vi "FTW-STR-Random-UTF8chars.vi"(3 "String Length":i32=32) -> (0 "Random UTF-8 Characters":string)   [LabVIEW 2013]
panel:
  out "Array 2":i32[](array[numeric])
  out "Numeric":i32
  out "Array":string[](array[string])
  out "x/y":dbl
  # "Inputs"
  # "Outputs"
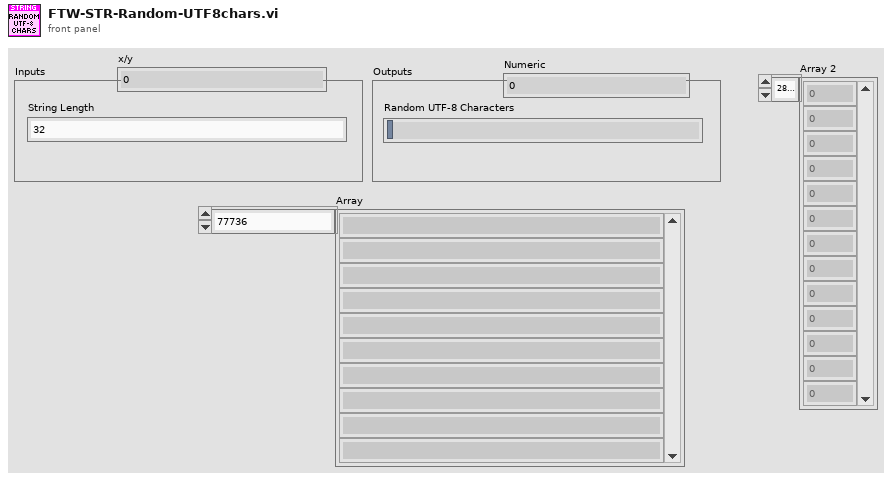
[diagram p1: front panel]
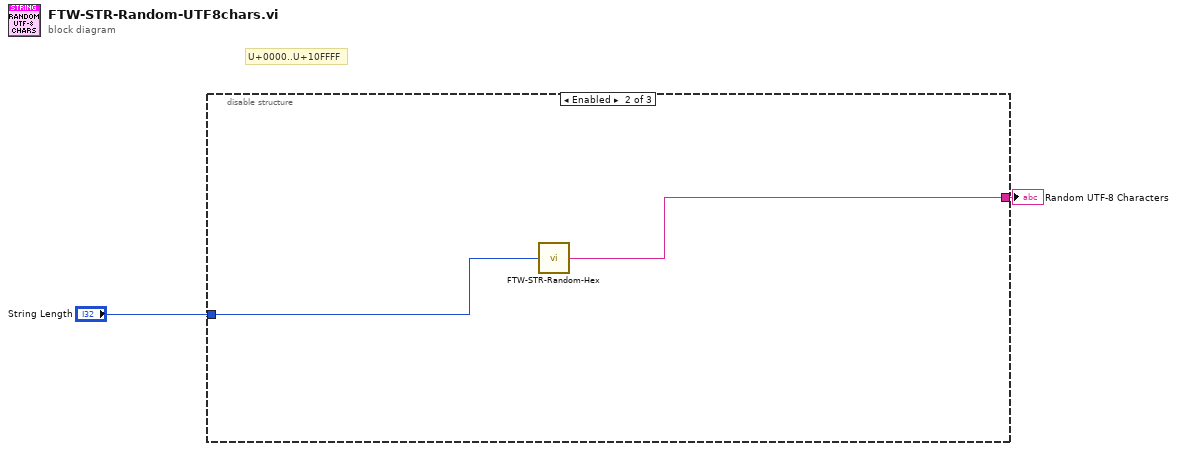
[diagram p0: block diagram]
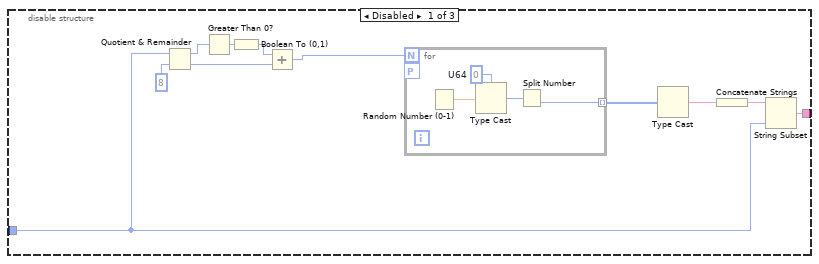
[diagram p2: hidden frame]
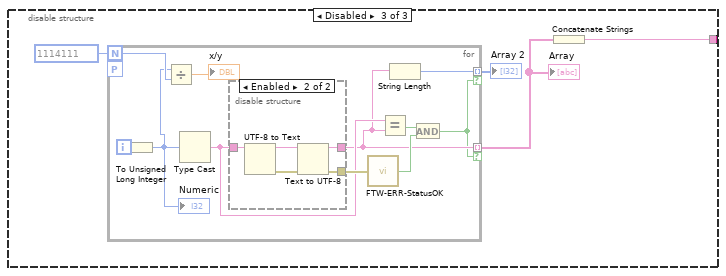
[diagram p3: hidden frame]
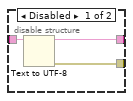
[diagram p4: hidden frame]
diagram:
  # "U+0000..U+10FFFF"
  n1 = disable-structure shown="Enabled" {
    disable-tunnel: [w13 w18 w21] -> w2
    disable-tunnel: "String Length" -> [w12 w19 _]
    frame Disabled {
      n2 = Quotient & Remainder(x=w12, y=8) -> (x-y*floor(x/y)=w9:i32, floor(x/y)=w6:i32)
      n3 = Greater Than 0?(x=w9) -> (x > 0?=w8:bool)
      n4 = Boolean To (0,1)(Boolean=w8) -> (0, 1=w7:i16)
      n5 = Add(x=w7, y=w6) -> (x+y=w5:i32)
      n6 = for {
        N: w5 -> [_]
        tunnel: [w14] -> w4 mode=indexing
        workers-P: _ -> [_]
        w16 = u64 0  # U64
        n7 = Random Number (0-1)() -> (number: 0 to 1=w17:dbl)
        n8 = Type Cast(type=w16, x=w17) -> (*(type *) &x=w15:u64)
        n9 = Split Number(x=w15) -> (lo(x)=w14:u32)  [unwired: 1 out]
      }
      n10 = Type Cast(x=w4) -> (*(type *) &x=w3:string)  [unwired: 1 in]
      n11 = Concatenate Strings(w3) -> (w10:string)
      n12 = String Subset(string=w10, length (rest)=w12) -> (substring=w13:string)  [unwired: 1 in]
    }
    frame Enabled {
      n13 = call "FTW-STR-Random-Hex.vi"("String Length"=w19) -> ("Random Hex String"=w18:string)  [unwired: 3 in]
    }
    frame Disabled {
      n14 = for {
        N: 1114111 -> [w33]
        tunnel: [w27] -> w22 mode=indexing if=w25
        workers-P: _ -> [_]
        tunnel: [w26] -> w20 mode=indexing if=w25
        i -> [w32]
        n15 = To Unsigned Long Integer(number=w32) -> (unsigned 32bit integer=w24:u32)
        "Numeric" <- w24
        n16 = Divide(x=w24, y=w33) -> (x/y=→"x/y":dbl)
        n17 = Type Cast(x=w24) -> (*(type *) &x=w30:string)  [unwired: 1 in]
        n18 = disable-structure shown="Enabled" {
          disable-tunnel: w30 -> [w37 w42]
          disable-tunnel: [w36 w38] -> w34
          disable-tunnel: [w35 w39] -> w27
          frame Disabled {
            n19 = Text to UTF-8(11:w37) -> (0:w36:errorcluster, 3:w35:string)  [unwired: 1 in]
          }
          frame Enabled {
            n20 = UTF-8 to Text(11:w42) -> (0:w40:errorcluster, 3:w41:string)  [unwired: 1 in]
            n21 = Text to UTF-8(8:w40, 11:w41) -> (0:w38:errorcluster, 3:w39:string)
          }
        }
        n22 = call "FTW-ERR-StatusOK.vi"("error to check"=w34) -> ("Status OK?"=w28:bool)
        n23 = Equal?(x=w30, y=w27) -> (x = y?=w29:bool)
        n24 = String Length(string=w27) -> (length=w26:i32)
        n25 = And(x=w29, y=w28) -> (x .and. y?=w25:bool)
      }
      "Array" <- w22
      "Array 2" <- w20
      n26 = Concatenate Strings(w22) -> (w21:string)
    }
  }
  "Random UTF-8 Characters" <- w2
